vi "PixelReg_presort.vi"(8 "EQ Data and Report":u32[](array[numeric])=[2137719168, 671965161, 2137719168, 671965161, 2137719168, 671965161, 2137719168, 671965161, 2137719168, 671965161, 2137719168, 671965161, 2137719168, 671965161, 2137719168, 671965161, 2137719168, 671965161, 2137719168, 671965161, 2137719168, 671965161, 2137719168, 671965161, 2137719168, 671965161, 2137719168, 671965161, 2137719168, 671965161, 2137719168, 671965161, 2137719168, 671965161, 2137719168, 671965161, 2137719168, 671965161, 2137719168, 671965161, 2137719168, 671965161, 2137719168, 671965161, 2137719168, 671965161, 2137719168, 671965161, 2137719168, 671965161, 2137719168, 671965161, 2137719168, 671965161, 2137719168, 671965161, 2137719168, 671965161, 2137719168, 671965161, 2137719168, 671965161, 2137719168, 671965161, 2137719168, 671965161, 2137719168, 671965161, 2137719168, 671965161, 2137719168, 671965161, 2137719168, 671965161, 2137719168, 671965161, 2137719168, 671965161, 2137719168, 671965161, 2137719168, 671965161, 2137719168, 671965161, 2137719168, 671965161, 2137719168, 671965161, 2137719168, 671965161, 2137719168, 760049897, 2137719168, 491616745, 2137719168, 671965161, 2137719168, 671965161, 2137719168, 671965161, 2137719168, 671965161, 2137719168, 671965161, 2137719168, 671965161, 2137719168, 671965161, 2137719168, 671965161, 2137719168, 671965161, 2137719168, 671965161, 2137719168, 671965161, 2137719168, 671965161, 2137719168, 671965161, 2137719168, 671965161, 2137719168, 671965161, 2137719168, 671965161, 2137719168, 671965161, 2137719168, 671965161, 2137719168, 671965161, 2137719168, 671965161, 2137719168, 671965161, 2137719168, 671965161, 2137719168, 671965161, 2137719168, 671965161, 2137719168, 671965161, 2137719168, 671965161, 2137719168, 671965161, 2137719168, 671965161, 2137719168, 671965161, 2137719168, 671965161, 2137719168, 671965161, 2137719168, 671965161, 2137719168, 671965161, 2137719168, 671965161, 2137719168, 671965161, 2137719168, 671965161, 2137719168, 671965161, 2137719168, 671965161, 2137719168, 671965161, 2137719168, 671965161, 2137719168, 671965161, 2137719168, 671965161, 2137719168, 671965161, 2137719168, 671965161, 2137719168, 671965161, 2137719168, 671965161, 2137719168, 671965161, 2137719168, 671965161, 2137719168, 671965161, 2137719168, 671965161, 2137719168, 671965161, 2137719168, 671965161, 2137719168, 671965161, 2070610304, 671965161, 2070610304, 671965161, 2070610304, 671965161, 2070610304, 671965161, 2070610304, 671965161, 2070610304, 671965161, 2070610304, 671965161, 2070610304, 671965161, 2070610304, 671965161, 2070610304, 671965161, 2070610304, 671965161, 2070610304, 671965161, 2070610304, 671965161, 2070610304, 671965161, 2070610304, 671965161, 2070610304, 671965161, 2070610304, 671965161, 2070610304, 671965161, 2070610304, 671965161, 2070610304, 671965161, 2070610304, 671965161, 2070610304, 671965161, 2070610304, 671965161, 2070610304, 671965161, 2070610304, 671965161, 2070610304, 671965161, 2070610304, 671965161, 2070610304, 671965161, 2070610304, 671965161, 2070610304, 671965161, 2070610304, 671965161, 2070610304, 671965161, 2070610304, 671965161, 2070610304, 671965161, 2070610304, 671965161, 2070610304, 671965161, 2070610304, 671965161, 2070610304, 671965161, 2070610304, 671965161, 2070610304, 671965161, 2070610304, 671965161, 2070610304, 671965161, 2070610304, 671965161, 2070610304, 671965161, 2070610304, 671965161, 2070610304, 891148969, 2070610304, 1223555977, 2070610304, 671965161, 2070610304, 671965161, 2070610304, 671965161, 2070610304, 671965161, 2070610304, 671965161, 2070610304, 671965161, 2070610304, 671965161, 2070610304, 671965161, 2070610304, 671965161, 2070610304, 671965161, 2070610304, 671965161, 2070610304, 671965161, 2070610304, 671965161, 2070610304, 671965161, 2070610304, 671965161, 2070610304, 671965161, 2070610304, 671965161, 2070610304, 671965161, 2070610304, 671965161, 2070610304, 671965161, 2070610304, 671965161, 2070610304, 671965161, 2070610304, 671965161, 2070610304, 671965161, 2070610304, 671965161, 2070610304, 671965161, 2070610304, 671965161, 2070610304, 671965161, 2070610304, 671965161, 2070610304, 671965161, 2070610304, 671965161, 2070610304, 671965161, 2070610304, 671965161, 2070610304, 671965161, 2070610304, 671965161, 2070610304, 671965161, 2070610304, 671965161, 2070610304, 671965161, 2070610304, 671965161, 2070610304, 671965161, 2070610304, 671965161, 2070610304, 671965161, 2070610304, 671965161, 2070610304, 671965161, 2070610304, 671965161, 2070610304, 671965161, 2070610304, 671965161, 2070610304, 671965161, 2070610304, 671965161, 2070610304, 671965161, 2070610304, 671965161, 2070610304, 671965161, 2070610304, 671965161, 2104164736, 671965161, 2104164736, 671965161, 2104164736, 671965161, 2104164736, 671965161, 2104164736, 671965161, 2104164736, 671965161, 2104164736, 671965161, 2104164736, 671965161, 2104164736, 671965161, 2104164736, 671965161, 2104164736, 671965161, 2104164736, 671965161, 2104164736, 671965161, 2104164736, 671965161, 2104164736, 671965161, 2104164736, 671965161, 2104164736, 671965161, 2104164736, 671965161, 2104164736, 671965161, 2104164736, 671965161, 2104164736, 671965161, 2104164736, 671965161, 2104164736, 671965161, 2104164736, 671965161, 2104164736, 671965161, 2104164736, 671965161, 2104164736, 671965161, 2104164736, 671965161, 2104164736, 671965161, 2104164736, 671965161, 2104164736, 671965161, 2104164736, 671965161, 2104164736, 671965161, 2104164736, 671965161, 2104164736, 671965161, 2104164736, 671965161, 2104164736, 671965161, 2104164736, 671965161, 2104164736, 671965161, 2104164736, 671965161, 2104164736, 671965161, 2104164736, 671965161, 2104164736, 671965161, 2104164736, 671965161, 2104164736, 671965161, 2104164736, 691900489, 2104164736, 960314249, 2104164736, 671965161, 2104164736, 671965161, 2104164736, 671965161, 2104164736, 671965161, 2104164736, 671965161, 2104164736, 671965161, 2104164736, 671965161, 2104164736, 671965161, 2104164736, 671965161, 2104164736, 671965161, 2104164736, 671965161, 2104164736, 671965161, 2104164736, 671965161, 2104164736, 671965161, 2104164736, 671965161, 2104164736, 671965161, 2104164736, 671965161, 2104164736, 671965161, 2104164736, 671965161, 2104164736, 671965161, 2104164736, 671965161, 2104164736, 671965161, 2104164736, 671965161, 2104164736, 671965161, 2104164736, 671965161, 2104164736, 671965161, 2104164736, 671965161, 2104164736, 671965161, 2104164736, 671965161, 2104164736, 671965161, 2104164736, 671965161, 2104164736, 671965161, 2104164736, 671965161, 2104164736, 671965161, 2104164736, 671965161, 2104164736, 671965161, 2104164736, 671965161, 2104164736, 671965161, 2104164736, 671965161, 2104164736, 671965161, 2104164736, 671965161, 2104164736, 671965161, 2104164736, 671965161, 2104164736, 671965161, 2104164736, 671965161, 2104164736, 671965161, 2104164736, 671965161, 2104164736, 671965161, 2104164736, 671965161, 2104164736, 671965161, 2104164736, 671965161, 2104164736, 671965161, 2104164736, 671965161, 2028667264, 671965161, 2028667264, 671965161, 2028667264, 671965161, 2028667264, 671965161, 2028667264, 671965161, 2028667264, 671965161, 2028667264, 671965161, 2028667264, 671965161, 2028667264, 671965161, 2028667264, 671965161, 2028667264, 671965161, 2028667264, 671965161, 2028667264, 671965161, 2028667264, 671965161, 2028667264, 671965161, 2028667264, 671965161, 2028667264, 671965161, 2028667264, 671965161, 2028667264, 671965161, 2028667264, 671965161, 2028667264, 671965161, 2028667264, 671965161, 2028667264, 671965161, 2028667264, 671965161, 2028667264, 671965161, 2028667264, 671965161, 2028667264, 671965161, 2028667264, 671965161, 2028667264, 671965161, 2028667264, 671965161, 2028667264, 671965161, 2028667264, 671965161, 2028667264, 671965161, 2028667264, 671965161, 2028667264, 671965161, 2028667264, 671965161, 2028667264, 671965161, 2028667264, 671965161, 2028667264, 671965161, 2028667264, 671965161, 2028667264, 671965161, 2028667264, 671965161, 2028667264, 671965161, 2028667264, 671965161, 2028667264, 671965161, 2028667264, 555604297, 2028667264, 689765225, 2028667264, 671965161, 2028667264, 671965161, 2028667264, 671965161, 2028667264, 671965161, 2028667264, 671965161, 2028667264, 671965161, 2028667264, 671965161, 2028667264, 671965161, 2028667264, 671965161, 2028667264, 671965161, 2028667264, 671965161, 2028667264, 671965161, 2028667264, 671965161, 2028667264, 671965161, 2028667264, 671965161, 2028667264, 671965161, 2028667264, 671965161, 2028667264, 671965161, 2028667264, 671965161, 2028667264, 671965161, 2028667264, 671965161, 2028667264, 671965161, 2028667264, 671965161, 2028667264, 671965161, 2028667264, 671965161, 2028667264, 671965161, 2028667264, 671965161, 2028667264, 671965161, 2028667264, 671965161, 2028667264, 671965161, 2028667264, 671965161, 2028667264, 671965161, 2028667264, 671965161, 2028667264, 671965161, 2028667264, 671965161, 2028667264, 671965161, 2028667264, 671965161, 2028667264, 671965161, 2028667264, 671965161, 2028667264, 671965161, 2028667264, 671965161, 2028667264, 671965161, 2028667264, 671965161, 2028667264, 671965161, 2028667264, 671965161, 2028667264, 671965161, 2028667264, 671965161, 2028667264, 671965161, 2028667264, 671965161, 2028667264, 671965161, 2028667264, 671965161, 2028667264, 671965161, 2028667264, 671965161, 0, 0, 0, 0, 2137719295, 4294967295, 4294967295, 4294967264, 235670073, 68228136, 2070610431, 4294967295, 4294967295, 4294967264, 235670073, 68228136, 2104164863, 4294967295, 4294967295, 4294967264, 235670073, 68228136, 2028667391, 4294967295, 4294967295, 4294967264, 235670073, 68228136, 2137718784, 4293787621, 59180718, 2137718785, 262139, 58525283, 2137718786, 58525283, 58525283, 2137718787, 58525283, 58525283, 2137718788, 58525283, 58525283, 2137718789, 58525283, 58525283, 2137718790, 58525283, 58525283, 2137718791, 58525283, 58525283] format="%x", 11 "Chip ID list":u32[](array[numeric]) format="%x") -> (1 "EQ Data and Report out":u32[](array[numeric]) format="%x")   [LabVIEW 2015, in "VIPM2.lvlib"]
doc: "Després de fer Program PixelRegister amb LayerID=FFFF, aquest subVI pre-endreça els PixelReg per Layers, per poder fer comprovacions i gravar arxius.\nManté l'ordre de Chip ID list."
uses:
  VIPM2.lvlib
panel:
  out "quants":i32[](array[numeric])
  out "Data+Report ordLayers":u32[][](array[numeric]) format="%x"
  # "Si Layer = FFFF, pre endreça les Layers per despres fer els Chip files"
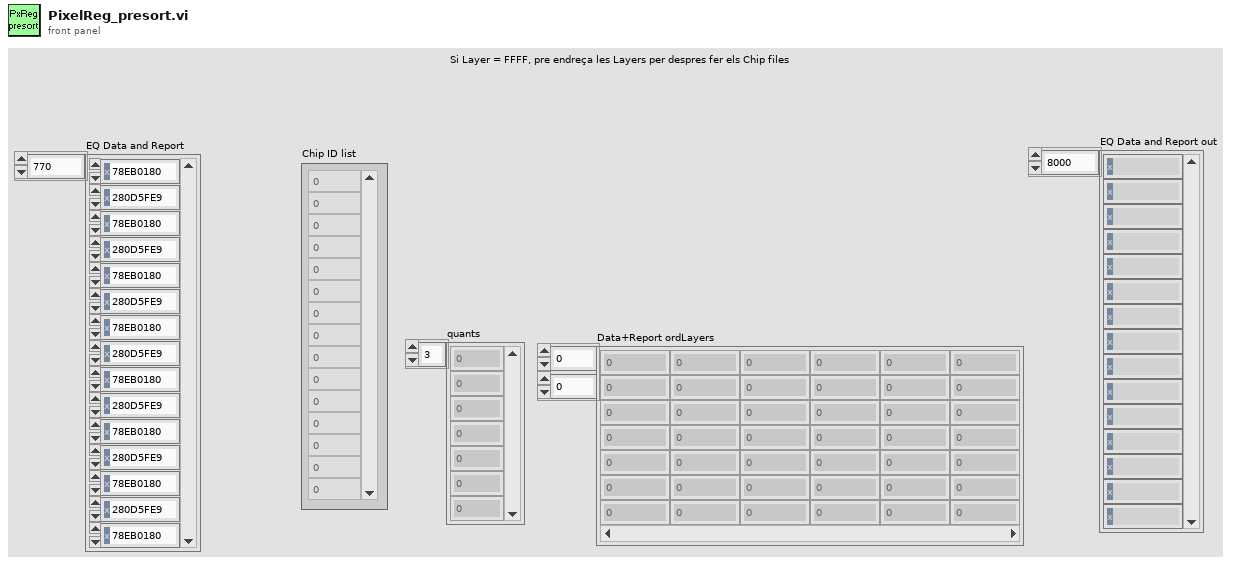
[diagram p1: front panel]
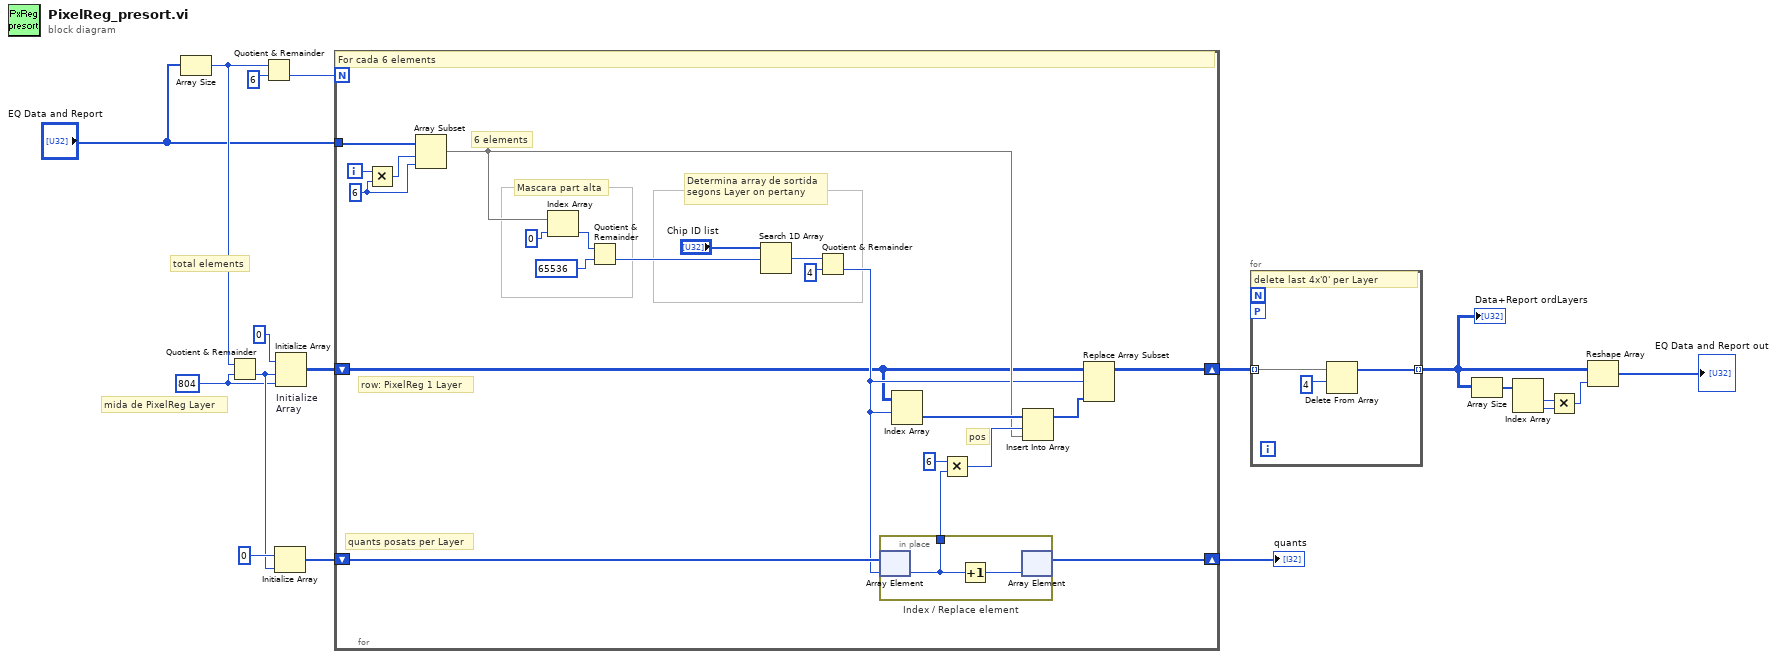
[diagram p0: block diagram]
diagram:
  w3 = 804 ("dimension size")
  # "mida de PixelReg Layer"
  # "total elements"
  n1 = Array Size(array="EQ Data and Report") -> (size(s)=w13:i32)
  n2 = Quotient & Remainder(x=w13, y=w3) -> (floor(x/y)=w10:i32)  [unwired: 1 out]
  n3 = Quotient & Remainder(x=w13, y=6) -> (floor(x/y)=w17:i32)  [unwired: 1 out]
  n4 = Initialize Array(0 ("y"), w10) -> (w12:i32[])
  n5 = Initialize Array "Initialize\nArray"(u32 0 ("dimension size"), w10, w3) -> (w15:u32[][])
  n6 = for {
    N: w17 -> [_]
    tunnel: "EQ Data and Report" -> [w39]
    shift-right: [w24] -> w1
    shift-left: w15 -> [w19]
    shift-right: [w20] -> w16
    shift-left: w12 -> [w23]
    i -> [w40]
    w37 = 6 ("y")
    # "row: PixelReg 1 Layer"
    # "pos"
    # "Determina array de sortida\nsegons Layer on pertany"
    # "quants posats per Layer"
    # "Mascara part alta"
    # "6 elements"
    # "For cada 6 elements"
    n7 = Multiply(x=w40, y=w37) -> (x*y=w38:i32)
    n8 = Array Subset "Array Subset"(array=w39, index=w38, length=w37) -> (w26:u32[])
    n9 = Index Array(array=w26, index=0) -> (element=w34:u32)
    n10 = Quotient & Remainder(x=w34, y=u32 65536) -> (floor(x/y)=w33:u32)  [unwired: 1 out]
    n11 = Search 1D Array(1D array="Chip ID list", element=w33) -> (index of element=w31:i32)  [unwired: 1 in]
    n12 = Quotient & Remainder(x=w31, y=4) -> (floor(x/y)=w22:i32)  [unwired: 1 out]
    n13 = in-place "Index / Replace element" {
      in-place-border: [w42] -> w21
      n14 = in-place-array #1(w23, w22) -> (w42:i32)
      n15 = Increment(x=w42) -> (x+1=w41:i32)
      n16 = in-place-array #1(w41) -> (w20:i32[])  [unwired: 1 out]
    }
    n17 = Index Array "Index Array"(array=w19, index (row)=w22) -> (element=w28:u32[])  [unwired: 1 in]
    n18 = Multiply(x=6, y=w21) -> (x*y=w27:i32)
    n19 = Insert Into Array "Insert Into Array"(array=w28, index=w27, new element=w26) -> (w25:u32[])
    n20 = Replace Array Subset "Replace Array Subset"(array=w19, new element=w25, index (row)=w22) -> (w24:u32[][])  [unwired: 1 in]
  }
  "quants" <- w16
  n21 = for {
    tunnel: w1 -> [w45] mode=indexing
    tunnel: [w43] -> w2 mode=indexing
    workers-P: _ -> [_]
    # "delete last 4x'0' per Layer"
    n22 = Delete From Array "Delete From Array"(array=w45, length=4) -> (array with subset deleted=w43:u32[])  [unwired: 1 in, 1 out]
  }
  "Data+Report ordLayers" <- w2
  n23 = Array Size(array=w2) -> (size(s)=w9:i32[])
  n24 = Index Array(array=w9) -> (element #1=w7:i32, element #2=w8:i32)  [unwired: 2 in]
  n25 = Multiply(x=w7, y=w8) -> (x*y=w6:i32)
  n26 = Reshape Array "Reshape Array"(w2, w6) -> (→"EQ Data and Report out":u32[])
